vi "IMAQ Preview the image Call Back.vi"() -> ()   [LabVIEW 2018]
uses:
  LabViewDVPCamera/LabViewDVPCamera.lvlib
panel:
  out "Image":T1(plugin-control)
  in  "EncoderBackwardCounter":dbl
  in  "EncoderForwardCounter":dbl
  in  "EncoderReset":bool
  in  "Encoder":dbl
  out "Capture frame rate":sgl
  out "Total frame rate":u32
  out "pFrameCount out":T2
  out "frame rate":dbl format="%#.5g"
  out "number":u64
  out "Millisecond timing value 3":u32
  in  "CloseFlg":i32
  out "handle":u32
  in  "CameraList":u16(ring) items=["MGS2000-H2-192.168.10.24", "MGV130-H2-192.168.10.83", "MGV231-H2-192.168.10.91", "MGV231M-H2-192.168.10.77", "MGV502M-H2-192.168.10.85", "MGV600-H2-192.168.10.78", "MGV600M-H2-192.168.10.52", "RGL4K3C-H-192.168.10.69", "XL874000006"]
  in  "Set":bool
  in  "Close":bool
  in  "Open":bool
  in  "ScanCamera":bool
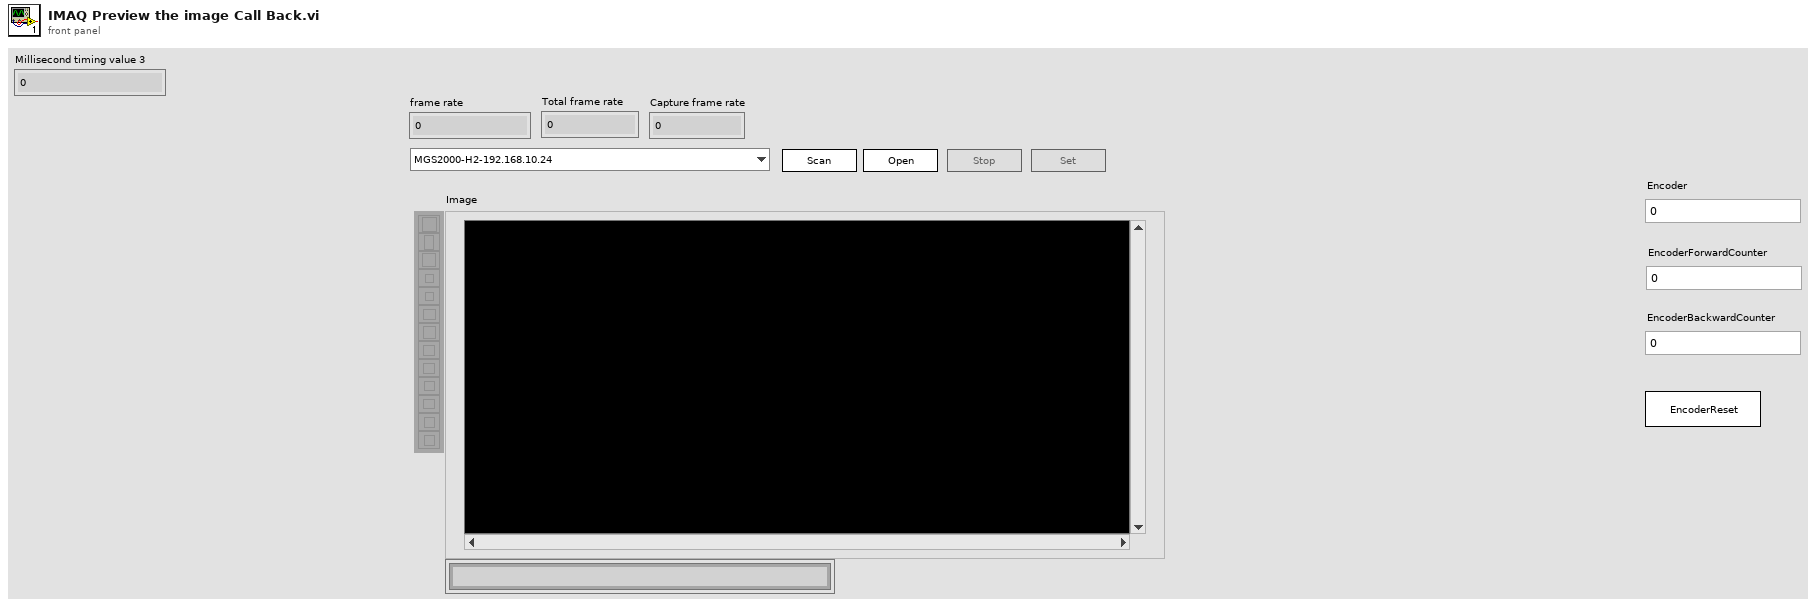
[diagram p1: front panel]
types:
  T1 = typedef "IMAQ Image.ctl" = refnum<image>
  T2 = cluster{"uFrameCount":u32, "uFrameDrop":u32, "uFrameIgnore":u32, "uFrameError":u32, "uFrameOK":u32, "uFrameOut":u32, "uFrameResend":u32, "uFrameProc":u32, "fFrameRate":sgl, "fProcRate":sgl, "reserved[0]":i32, "reserved[1]":i32, "reserved[2]":i32, "reserved[3]":i32, "reserved[4]":i32, "reserved[5]":i32, "reserved[6]":i32, "reserved[7]":i32, "reserved[8]":i32, "reserved[9]":i32, "reserved[10]":i32, "reserved[11]":i32, "reserved[12]":i32, "reserved[13]":i32, "reserved[14]":i32, "reserved[15]":i32, "reserved[16]":i32, "reserved[17]":i32, "reserved[18]":i32, "reserved[19]":i32, "reserved[20]":i32, "reserved[21]":i32, "reserved[22]":i32, "reserved[23]":i32, "reserved[24]":i32, "reserved[25]":i32, "reserved[26]":i32, "reserved[27]":i32, "reserved[28]":i32, "reserved[29]":i32, "reserved[30]":i32, "reserved[31]":i32}
  T3 = enum8{"Enabled", "Disabled", "Disabled and Grayed Out"}
  T4 = typedef "LVStringsAndValuesArrayTypeDef_U16.ctl" = cluster{"String":string, "Value":u16}[]
  T5 = typedef "Image Type" = u32
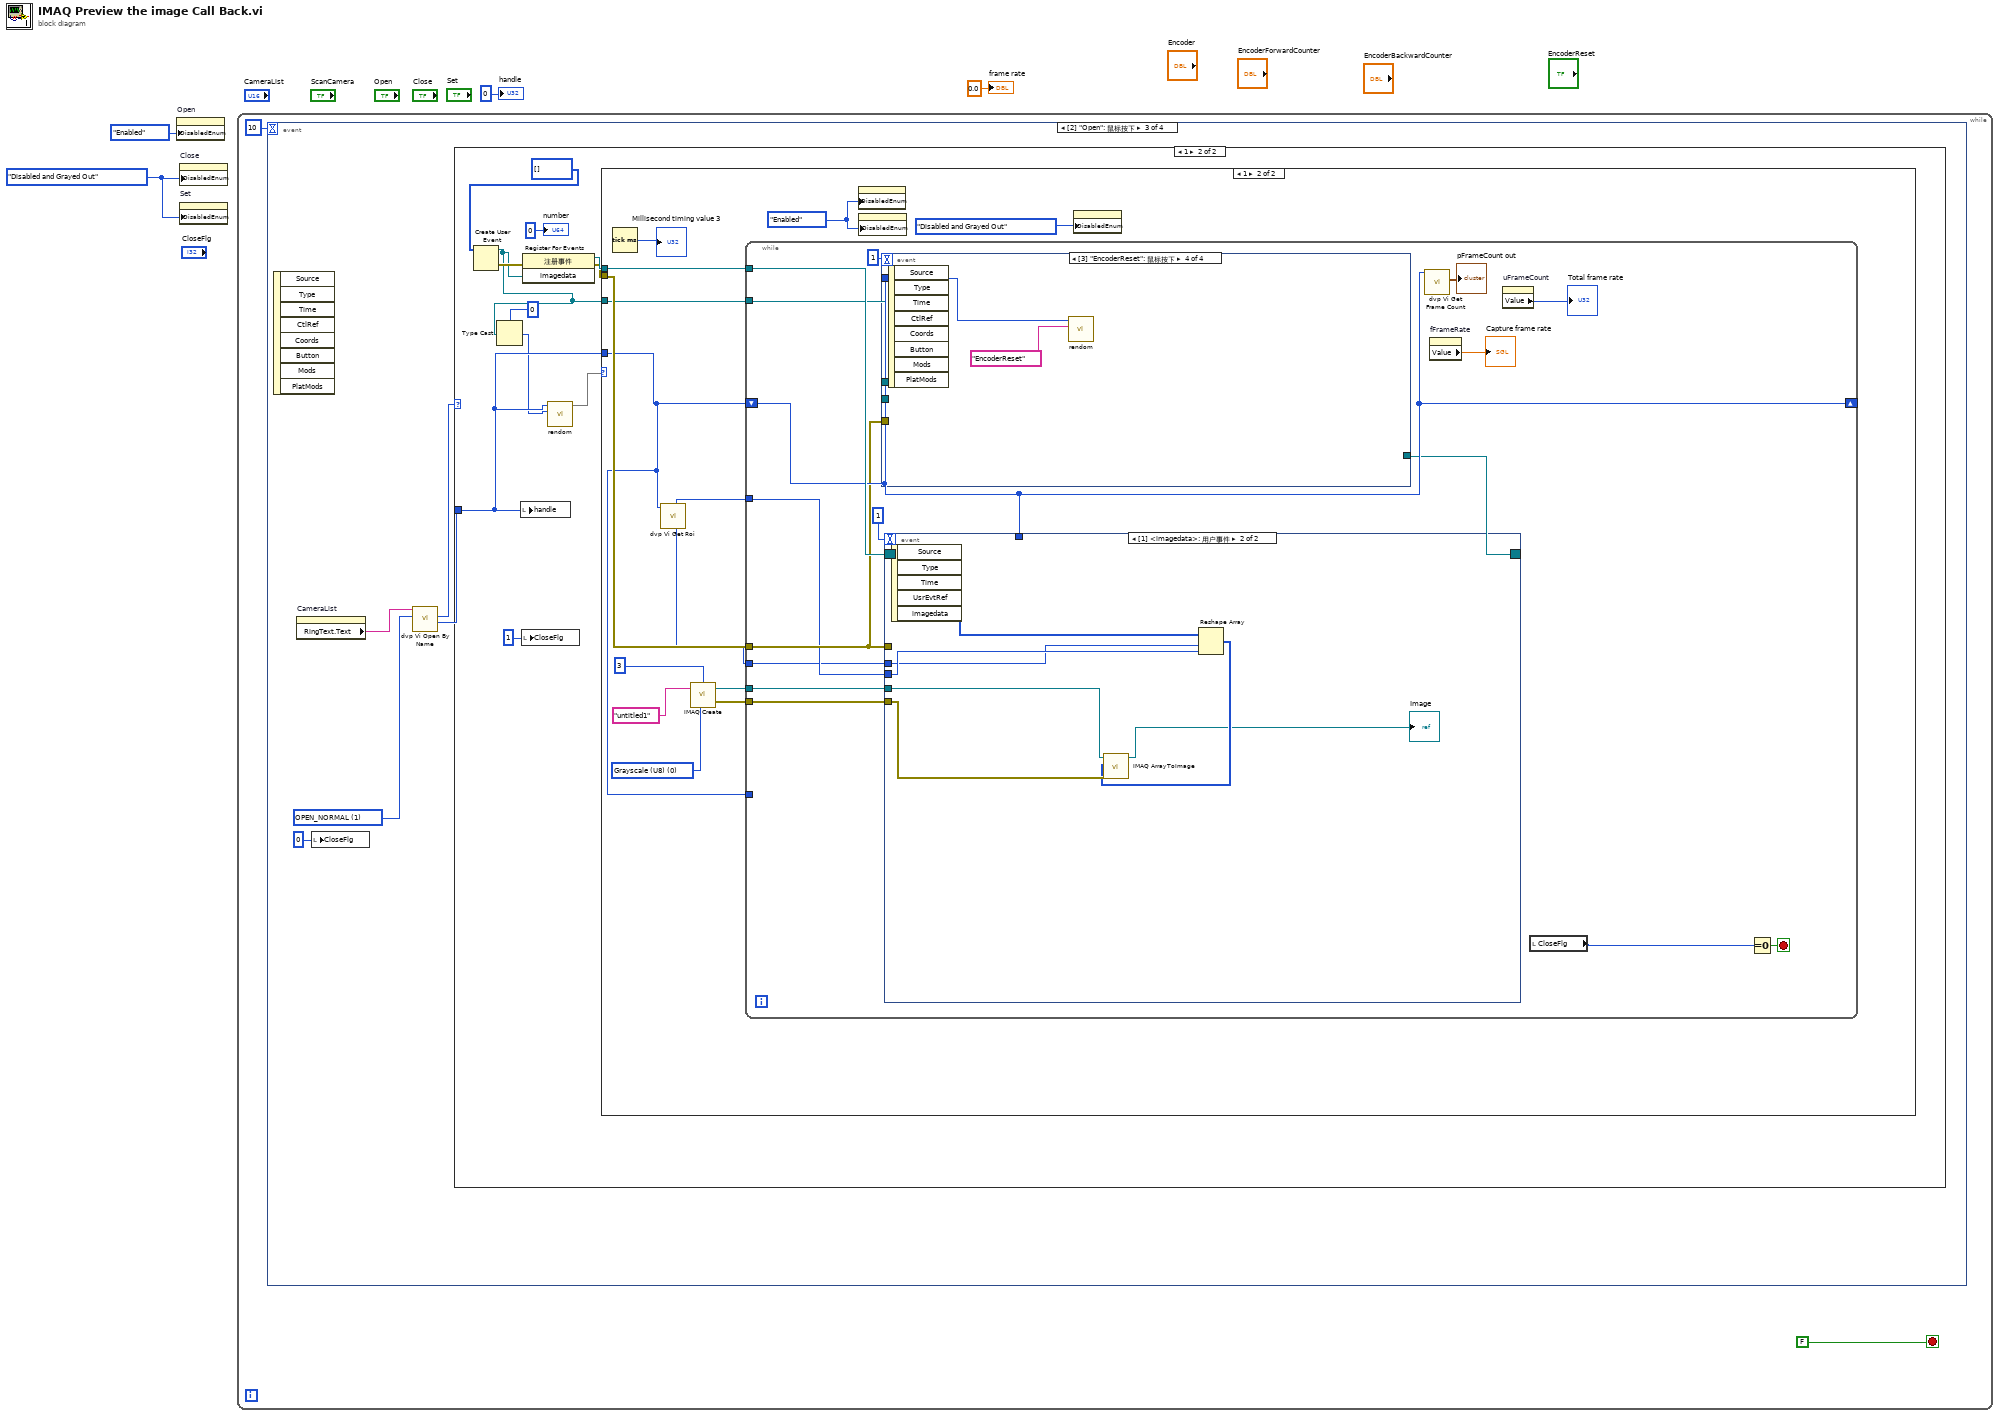
[diagram p0: block diagram]
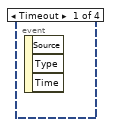
[diagram p2: hidden frame]
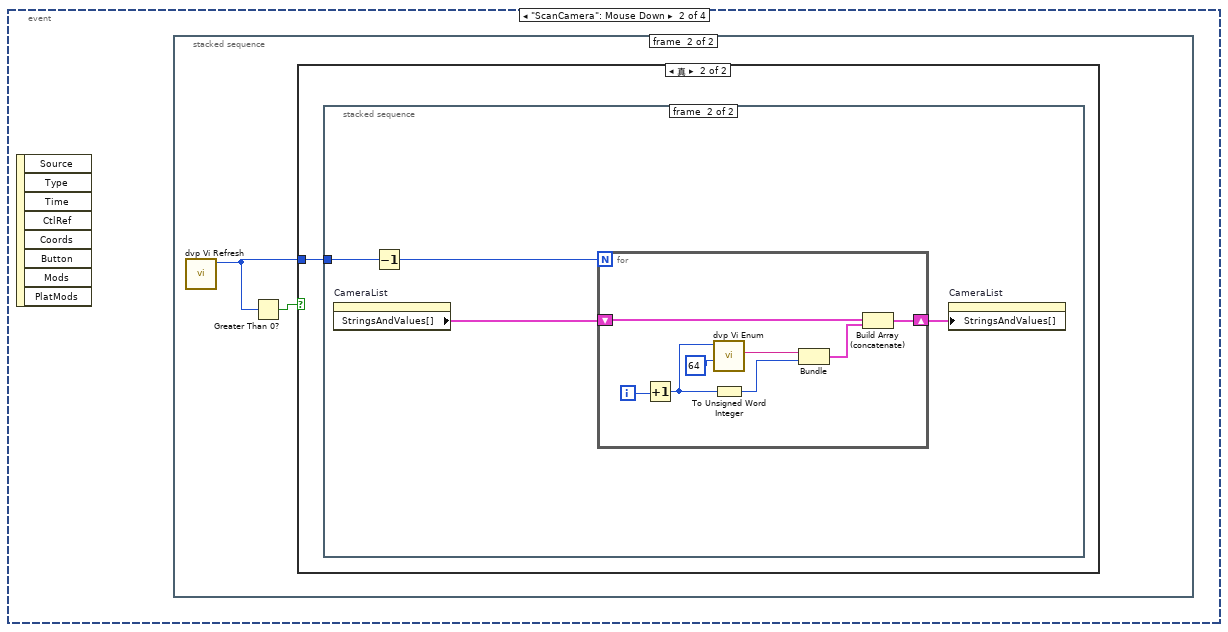
[diagram p3: hidden frame]
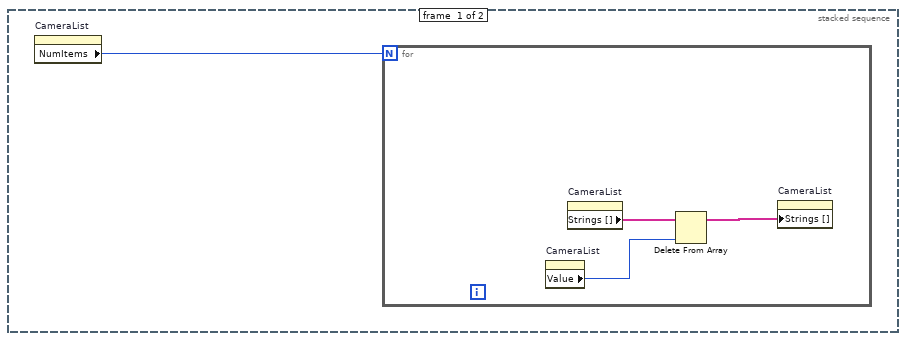
[diagram p4: hidden frame]
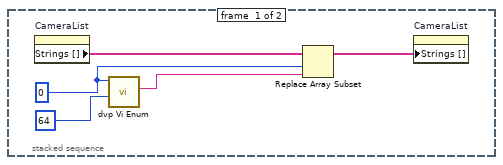
[diagram p6: hidden frame]
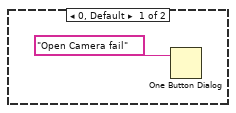
[diagram p7: hidden frame]
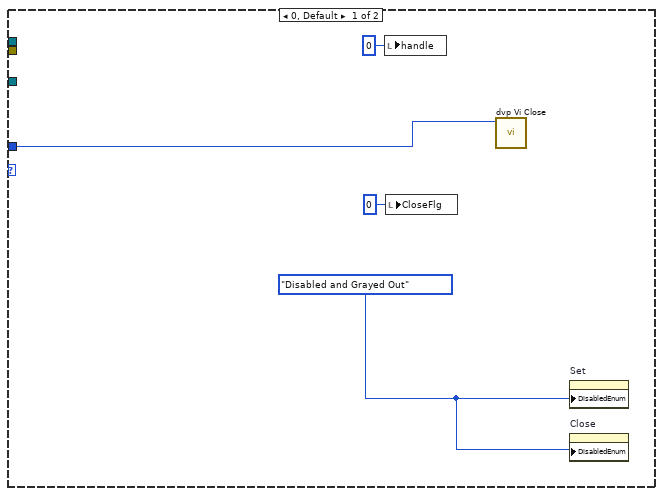
[diagram p8: hidden frame]
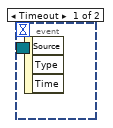
[diagram p9: hidden frame]
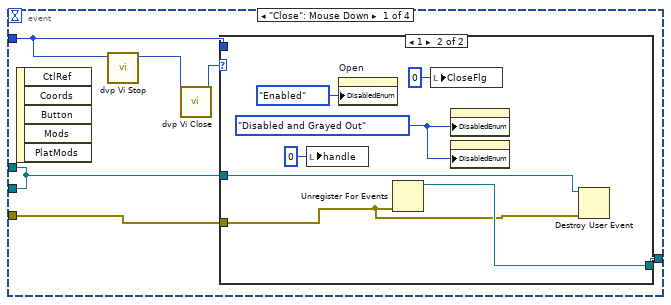
[diagram p10: hidden frame]
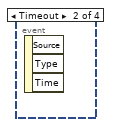
[diagram p12: hidden frame]
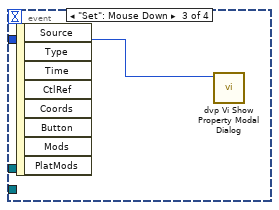
[diagram p13: hidden frame]
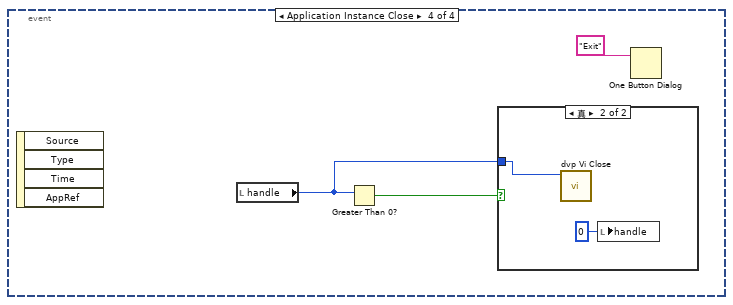
[diagram p14: hidden frame]
diagram:
  w3 = T3."Disabled and Grayed Out" ("禁用")
  n1 = property on="Open" class="Bool"("DisabledEnum"=T3."Enabled" ("禁用")) -> ()  [unwired: 2 in, 2 out]
  n2 = property on="Close" class="Bool"("DisabledEnum"=w3) -> ()  [unwired: 2 in, 2 out]
  n3 = property on="Set" class="Bool"("DisabledEnum"=w3) -> ()  [unwired: 2 in, 2 out]
  n4 = while {
    stop <- FALSE stop-if-true
    n5 = event shown="[2] \"Open\": 鼠标按下" {
      selector: _ -> [_ _ _ _]
      dyn-events: _ -> [_ _ _ _]
      timeout: 10 -> [_ _ _ _]
      event Timeout {
        n6 = event-data() -> ()  [unwired: 1 in, 3 out]
      }
      event "ScanCamera": Mouse Down {
        n7 = event-data() -> ()  [unwired: 1 in, 8 out]
        n8 = stacked-sequence "清除下拉列表的数据" {
          frame #0 {
            n9 = property on="CameraList" class="Ring (严格)"() -> ("NumItems"=w7:u32)  [unwired: 2 in, 2 out]
            n10 = for {
              N: w7 -> [_]
              n11 = property on="CameraList" class="Ring (严格)"() -> ("Value"=w9:u16)  [unwired: 2 in, 2 out]
              n12 = property on="CameraList" class="Ring (严格)"() -> ("Strings []"=w8:string[])  [unwired: 2 in, 2 out]
              n13 = Delete From Array ("删除数组元素")(array=w8, index=w9) -> (array with subset deleted=w10:string[])  [unwired: 1 in, 1 out]
              n14 = property on="CameraList" class="Ring (严格)"("Strings []"=w10) -> ()  [unwired: 2 in, 2 out]
            }
          }
          frame #1 {
            n15 = call "dvp Vi Refresh.vi"() -> ("pCount out"=w12:u32)  [unwired: 10 in, 1 out]
            n16 = Greater Than 0?(x=w12) -> (x > 0?=w11:bool)
            n17 = case shown="真" w11 {
              tunnel: w12 -> [_ w13]
              frame False {
              }
              frame True {
                n18 = stacked-sequence {
                  tunnel: w13 -> [_ w20]
                  frame #0 {
                    w14 = u32 0 ("index")
                    n19 = property on="CameraList" class="Ring (严格)"() -> ("Strings []"=w17:string[])  [unwired: 2 in, 2 out]
                    n20 = call "dvp Vi Enum.vi"("unSize"=u32 64, "index"=w14) -> ("friendlyName out"=w16:string)  [unwired: 8 in, 1 out]
                    n21 = Replace Array Subset ("替换数组子集")(array=w17, new element=w16, index=w14) -> (w18:string[])
                    n22 = property on="CameraList" class="Ring (严格)"("Strings []"=w18) -> ()  [unwired: 2 in, 2 out]
                  }
                  frame #1 {
                    n23 = property on="CameraList" class="Ring (严格)"() -> ("StringsAndValues[]"=w22:T4)  [unwired: 2 in, 2 out]
                    n24 = Decrement(x=w20) -> (x-1=w19:u32)
                    n25 = for {
                      N: w19 -> [_]
                      shift-right: [w29] -> w21
                      shift-left: w22 -> [w27]
                      i -> [w24]
                      n26 = Increment(x=w24) -> (x+1=w23:i32)
                      n27 = call "dvp Vi Enum.vi"("unSize"=u32 64, "index"=w23) -> ("friendlyName out"=w30:string)  [unwired: 8 in, 1 out]
                      n28 = To Unsigned Word Integer(number=w23) -> (unsigned 16bit integer=w26:u16)
                      n29 = Bundle("friendlyName out"=w30, w26) -> (w28:cluster{"friendlyName out":string, u16})  [unwired: 1 in]
                      n30 = Build Array (concatenate) ("创建数组")(w27, w28) -> (w29:T4)
                    }
                    n31 = property on="CameraList" class="Ring (严格)"("StringsAndValues[]"=w21) -> ()  [unwired: 2 in, 2 out]
                  }
                }
              }
            }
          }
        }
      }
      event "Open": Mouse Down {
        w33 = u32 1 items=["OPEN_OFFLINE", "OPEN_NORMAL"] ("type")
        n32 = event-data() -> ()  [unwired: 1 in, 8 out]
        n33 = property on="CameraList" class="Ring (严格)"() -> ("RingText.Text"=w32:string)  [unwired: 2 in, 2 out]
        n34 = local write "CloseFlg"(0 ("CloseFlg")) -> ()
        n35 = call "dvp Vi Open By Name.vi"("type"=w33, "friendlyName"=w32) -> ("pHandle out"=w35:u32, "function return"=w34:u32)  [unwired: 7 in, 1 out]
        n36 = case shown="1" w34 {
          tunnel: w35 -> [_ w40]
          frame 0, Default {
            n37 = One Button Dialog(message="Open Camera fail" ("消息")) -> ()  [unwired: 1 in, 1 out]
          }
          frame 1 {
            n38 = Create User Event(user event datatype=u8[] [] ("imagedata")) -> (user event=w41:refnum<user-event>, error out=w45:errorcluster)  [unwired: 1 in]
            n39 = Type Cast(type=0, x=w41) -> (*(type *) &x=w39:i32)
            n40 = local write "handle"(w40) -> ()
            n41 = local write "CloseFlg"(1 ("CloseFlg")) -> ()
            n42 = register-events(error in=w45, w41) -> (reference out=w43:refnum<event-registration>, error out=w42:errorcluster)  [unwired: 1 in]
            n43 = call "rendom.vi"("min"=w39, "max"=w40) -> (3:w38)  [unwired: 8 in, 1 out]
            n44 = case shown="1" w38 {
              tunnel: w40 -> [w51 w52]
              tunnel: w43 -> [_ w62]
              tunnel: w42 -> [_ w61]
              tunnel: w41 -> [_ w55]
              frame 0, Default {
                w50 = T3."Disabled and Grayed Out" ("禁用")
                n45 = local write "handle"(u32 0 ("handle")) -> ()
                n46 = local write "CloseFlg"(0 ("CloseFlg")) -> ()
                n47 = call "dvp Vi Close.vi"("handle"=w51) -> ()  [unwired: 10 in, 1 out]
                n48 = property on="Set" class="Bool"("DisabledEnum"=w50) -> ()  [unwired: 2 in, 2 out]
                n49 = property on="Close" class="Bool"("DisabledEnum"=w50) -> ()  [unwired: 2 in, 2 out]
              }
              frame 1 {
                w60 = T5 0 items=["Grayscale (U8)", "Grayscale (I16)", "Grayscale (SGL)", "Complex (CSG)", "RGB (U32)", "HSL (U32)", "RGB (U64)", "Grayscale (U16)"] ("Image Type")
                w65 = T3."Enabled" ("禁用")
                n50 = Tick Count (ms)() -> (millisecond timer value=→"Millisecond timing value 3":u32)
                n51 = call "dvp Vi Get Roi.vi"("handle"=w52) -> ("pH out"=w53:i32, "pW out"=w54:i32)  [unwired: 6 in, 3 out]
                n52 = call "IMAQ Create"("Border Size"=3, "Image Name"="untitled1", "Image Type"=w60) -> ("New Image"=w57:T1, "error out"=w56:errorcluster)  [unwired: 2 in]
                n53 = while {
                  shift-right: [w73] -> _
                  shift-left: w52 -> [w73]
                  tunnel: w62 -> [w75]
                  tunnel: w61 -> [w69]
                  tunnel: w57 -> [w72]
                  tunnel: w56 -> [w71]
                  tunnel: w55 -> [w68]
                  tunnel: w54 -> [w67]
                  tunnel: w53 -> [w66]
                  tunnel: w52 -> [_]
                  stop <- w80 stop-if-true
                  n54 = event shown="[1] <imagedata>: 用户事件" {
                    selector: w75 -> [_ _]
                    dyn-events: [_ _] -> w70
                    timeout: 1 -> [_ _]
                    tunnel: w69 -> [_ _]
                    tunnel: w73 -> [_ _]
                    tunnel: w72 -> [_ w84]
                    tunnel: w71 -> [_ w85]
                    tunnel: w67 -> [_ w87]
                    tunnel: w66 -> [_ w86]
                    event Timeout {
                      n55 = event-data() -> ()  [unwired: 1 in, 3 out]
                    }
                    event User Event {
                      n56 = event-data() -> ("imagedata"=w88:u8[])  [unwired: 1 in, 4 out]
                      n57 = Reshape Array ("重排数组维数")(w88, w86, w87) -> (w83:u8[][])
                      n58 = call "IMAQ ArrayToImage"("error in (no error)"=w85, "Image Pixels (U8)"=w83, "Image"=w84) -> ("Image Out"=→"Image":T1)  [unwired: 7 in, 1 out]
                    }
                  }
                  n59 = event shown="[3] \"EncoderReset\": 鼠标按下" {
                    selector: _ -> [_ _ _ _]
                    dyn-events: _ -> [_ _ _ _]
                    timeout: 1 -> [_ _ _ _]
                    tunnel: w73 -> [w90 _ w101 w103]
                    tunnel: w70 -> [w93 _ _ _]
                    tunnel: w69 -> [w92 _ _ _]
                    tunnel: [w91 _ _ _] -> _
                    tunnel: w68 -> [w91 _ _ _]
                    event "Close": Mouse Down {
                      n60 = event-data() -> ()  [unwired: 1 in, 5 out]
                      n61 = call "dvp Vi Stop.vi"("handle"=w90) -> ()  [unwired: 10 in, 1 out]
                      n62 = call "dvp Vi Close.vi"("handle"=w90) -> ("function return"=w89:u32)  [unwired: 10 in]
                      n63 = case shown="1" w89 {
                        tunnel: w90 -> [_ _]
                        tunnel: w93 -> [_ w96]
                        tunnel: w92 -> [_ w95]
                        tunnel: w91 -> [_ w94]
                        frame 0, Default {
                        }
                        frame 1 {
                          w98 = T3."Disabled and Grayed Out" ("禁用")
                          n64 = local write "handle"(u32 0 ("handle")) -> ()
                          n65 = property on="Open" class="Bool"("DisabledEnum"=T3."Enabled" ("禁用")) -> ()  [unwired: 2 in, 2 out]
                          n66 = Unregister For Events(event registration refnum=w96, error in=w95) -> ()  [unwired: 1 out]
                          n67 = local write "CloseFlg"(0 ("CloseFlg")) -> ()
                          n68 = property on="Close" class="Bool"("DisabledEnum"=w98) -> ()  [unwired: 2 in, 2 out]
                          n69 = property on="Set" class="Bool"("DisabledEnum"=w98) -> ()  [unwired: 2 in, 2 out]
                          n70 = Destroy User Event(user event=w94, error in=w95) -> ()  [unwired: 1 out]
                        }
                      }
                    }
                    event Timeout {
                      n71 = event-data() -> ()  [unwired: 1 in, 3 out]
                    }
                    event "Set": Mouse Down {
                      n72 = event-data() -> ()  [unwired: 1 in, 8 out]
                      n73 = call "dvp Vi Show Property Modal Dialog.vi"("handle"=w101) -> ()  [unwired: 10 in, 1 out]
                    }
                    event "EncoderReset": Mouse Down {
                      n74 = event-data() -> ()  [unwired: 1 in, 8 out]
                      n75 = call "rendom.vi"("min"="EncoderReset" ("Image Name"), "max"=w103) -> ()  [unwired: 9 in, 1 out]
                    }
                  }
                  n76 = call "dvp Vi Get Frame Count.vi"("handle"=w73) -> ("pFrameCount out"=→"pFrameCount out":T2)  [unwired: 9 in, 1 out]
                  n77 = property on="fFrameRate" class="DigNum (严格)"() -> ("Value"=→"Capture frame rate":sgl)  [unwired: 2 in, 2 out]
                  n78 = property on="uFrameCount" class="DigNum (严格)"() -> ("Value"=→"Total frame rate":u32)  [unwired: 2 in, 2 out]
                  n79 = local read "CloseFlg"() -> (w79:i32)
                  n80 = Equal To 0?(x=w79) -> (x = 0?=w80:bool)
                }
                n81 = property on="Set" class="Bool"("DisabledEnum"=w65) -> ()  [unwired: 2 in, 2 out]
                n82 = property on="Close" class="Bool"("DisabledEnum"=w65) -> ()  [unwired: 2 in, 2 out]
                n83 = property on="Open" class="Bool"("DisabledEnum"=T3."Disabled and Grayed Out" ("禁用")) -> ()  [unwired: 2 in, 2 out]
              }
            }
            "number" <- u64 0 ("数值")
          }
        }
      }
      event Application Instance Close {
        n84 = event-data() -> ()  [unwired: 1 in, 4 out]
        n85 = local read "handle"() -> (w104:u32)
        n86 = Greater Than 0?(x=w104) -> (x > 0?=w105:bool)
        n87 = case shown="真" w105 {
          tunnel: w104 -> [_ w108]
          frame False {
          }
          frame True {
            n88 = call "dvp Vi Close.vi"("handle"=w108) -> ()  [unwired: 10 in, 1 out]
            n89 = local write "handle"(u32 0 ("handle")) -> ()
          }
        }
        n90 = One Button Dialog(message="Exit" ("消息")) -> ()  [unwired: 1 in, 1 out]
      }
    }
  }
  "handle" <- u32 0 ("handle")
  "frame rate" <- 0.0 ("帧率")
